vi "Temperature Warnings.vi"(8 "Error In":errorcluster, 9 "Min Temperature":dbl, 10 "Max Temperature":dbl, 11 "Current Temperature":dbl) -> (0 "Error Out":errorcluster, 2 "Warning?":bool, 3 "Warning Text":string="No Warning")   [LabVIEW 2015]
doc: "This VI is used to determine the string to output to the weather station based on the current temperature and limit settings.\n\nInputs: Current Temperature (DBL), Minimum Temperature (DBL), and Maximum Temperature (DBL).\nOutputs: Warning Text (string) and Warning? (Boolean)."
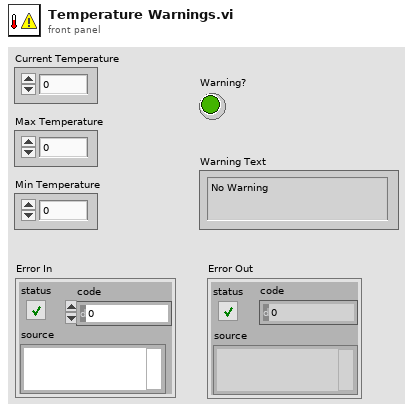
[diagram p1: front panel]
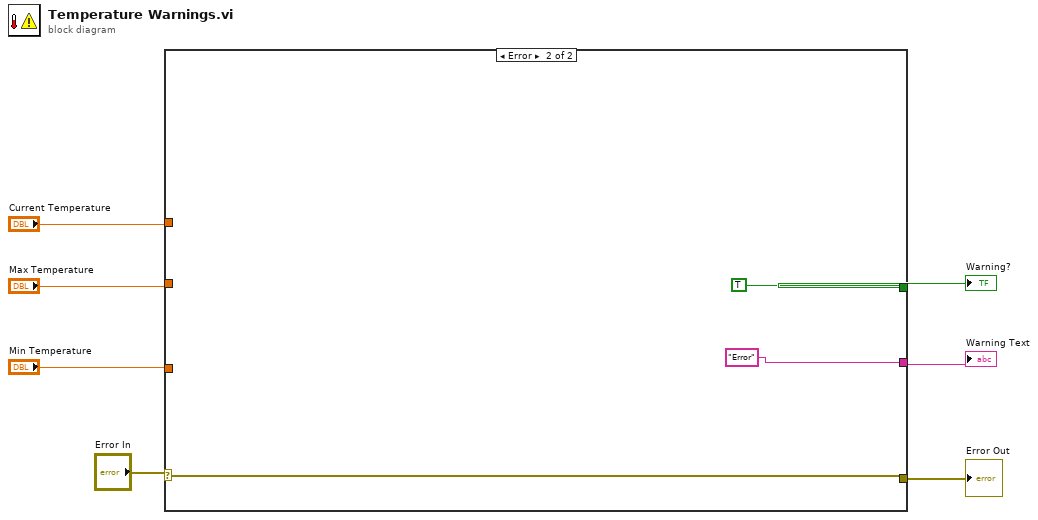
[diagram p0: block diagram]
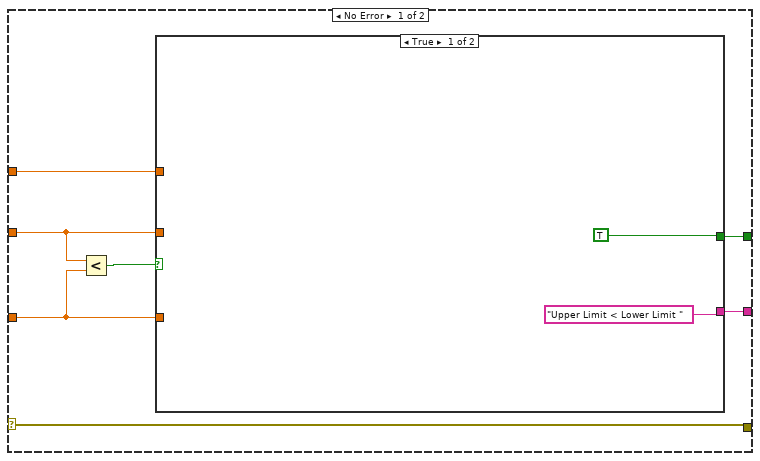
[diagram p2: hidden frame]
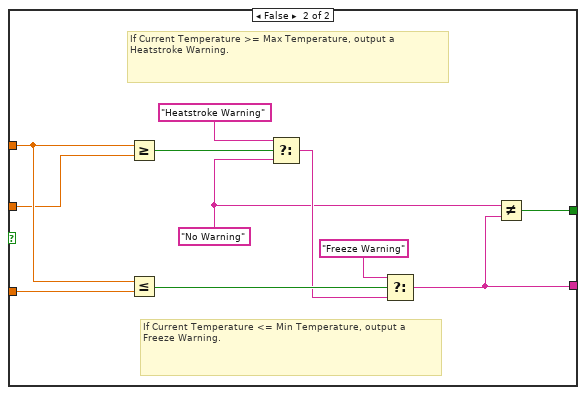
[diagram p3: hidden frame]
diagram:
  n1 = case shown="Error" "Error In" {
    selector: "Error In" -> [w8 w28]
    tunnel: "Current Temperature" -> [w14 _]
    tunnel: "Min Temperature" -> [w10 _]
    tunnel: "Max Temperature" -> [w11 _]
    tunnel: [w13 TRUE] -> w4
    tunnel: [w12 "Error"] -> w3
    tunnel: [w8 w28] -> w2
    frame No Error {
      n2 = Less?(x=w11, y=w10) -> (x < y?=w9:bool)
      n3 = case shown="True" w9 {
        tunnel: w14 -> [_ w27]
        tunnel: w10 -> [_ w26]
        tunnel: w11 -> [_ w25]
        tunnel: [TRUE w24] -> w13
        tunnel: ["Upper Limit < Lower Limit " w23] -> w12
        frame True {
        }
        frame False {
          w17 = "No Warning" ("f")
          # "If Current Temperature <= Min Temperature, output a Freeze Warning."
          # "If Current Temperature >= Max Temperature, output a Heatstroke Warning."
          n4 = Greater Or Equal?(x=w27, y=w25) -> (x >= y?=w22:bool)
          n5 = Less Or Equal?(x=w27, y=w26) -> (x <= y?=w19:bool)
          n6 = Select(t="Heatstroke Warning", s=w22, f=w17) -> (s? t:f=w18:string)
          n7 = Select(t="Freeze Warning", s=w19, f=w18) -> (s? t:f=w23:string)
          n8 = Not Equal?(x=w17, y=w23) -> (x != y?=w24:bool)
        }
      }
    }
    frame Error {
    }
  }
  "Warning?" <- w4
  "Warning Text" <- w3
  "Error Out" <- w2
